vi "CR-导丝颗粒物检测2处理函数.vi"(0 "Image in":T1(plugin-control), 9 "颗粒物个数阈值":i32, 11 "error in (no error)":errorcluster caption="错误输入（无错误）") -> (4 "Image out":T1(plugin-control), 6 "颗粒物有无显示":bool, 8 "颗粒物大小显示":dbl[](array[numeric]), 10 "颗粒物位置坐标":cluster{"X":dbl, "Y":dbl}[](array[cluster]) {"Y" format="%.2f"; "X" format="%.2f"}, 14 "Number of Features Found":i32, 15 "error out":errorcluster caption="错误输出")   [LabVIEW 2017]
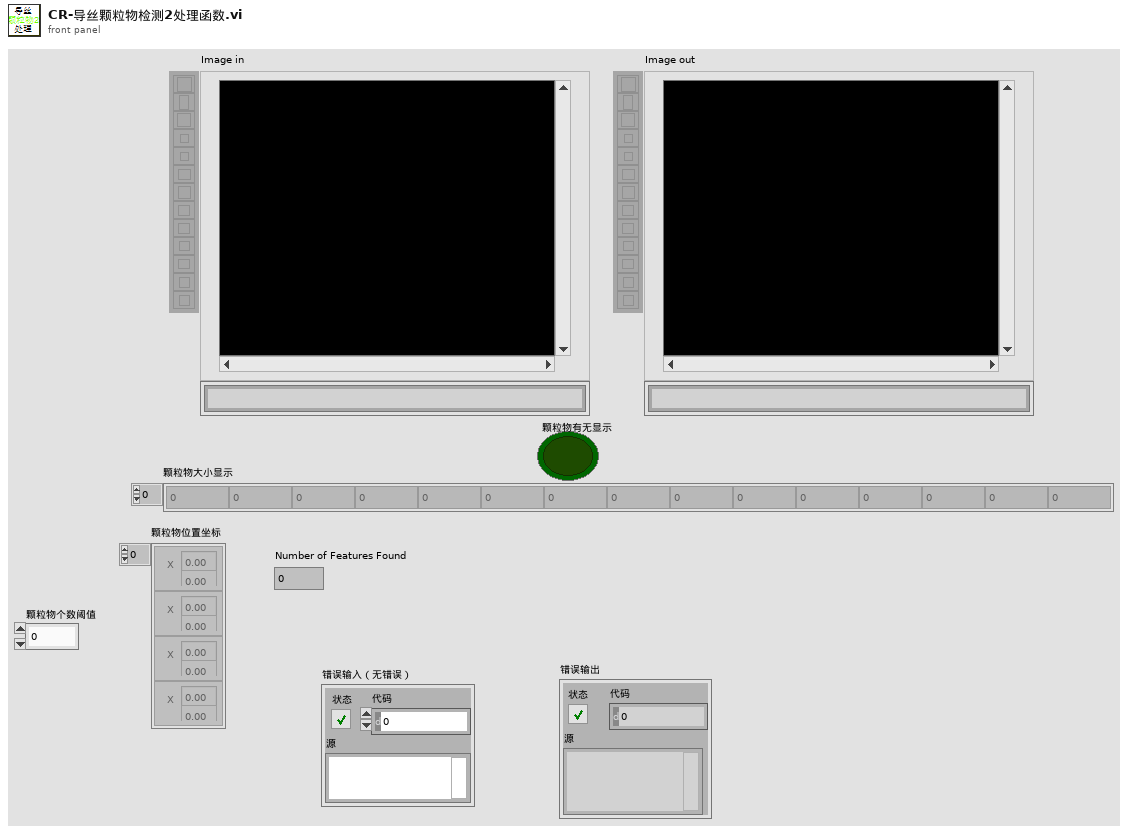
[diagram p1: front panel]
types:
  T1 = typedef "IMAQ Image.ctl" = refnum<image>
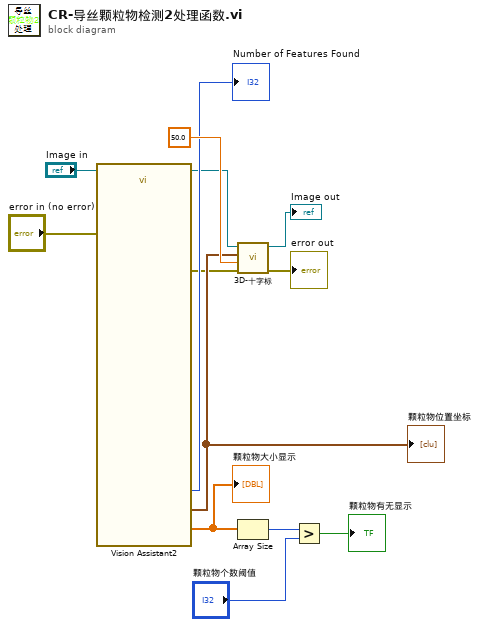
[diagram p0: block diagram]
diagram:
  n1 = call "Vision Assistant2"("Image In"="Image in", "error in"="error in (no error)") -> ("Image Out"=w3:T1, "Feature Points Strength (Feature Detection 1)"=w6:dbl[], "Number of Features Found (Feature Detection 1)"=→"Number of Features Found":i32, "Feature Points Coordinates (Feature Detection 1)"=w5:cluster{"X":dbl, "Y":dbl}[], "error out"=w4:errorcluster)  [unwired: 21 in]
  "颗粒物大小显示" <- w6
  "颗粒物位置坐标" <- w5
  n2 = call "3D-十字标.vi"("error in (no error)"=w4, "radius"=50.0, "颗粒物位置坐标"=w5, "输入图片"=w3) -> ("error out"=→"error out":errorcluster, "输出图片"=→"Image out":T1)  [unwired: 6 in]
  n3 = Array Size(array=w6) -> (size(s)=w13:i32)
  n4 = Greater?(x=w13, y="颗粒物个数阈值") -> (0:→"颗粒物有无显示":bool)
